vi "FetchIndividualElement.vi"() -> ()   [LabVIEW 2019]
uses:
  <vilib>/addons/database/Auxilliary.llb/DB Tools Cursor Type.ctl
  <vilib>/addons/database/Connection.llb/DB Tools Open Connec (String).vi
  <vilib>/addons/database/Connection.llb/Conn Execute.vi
  <vilib>/addons/database/Recordset.llb/Rec Fetch Integer Data (R).vi
  <vilib>/addons/database/Recordset.llb/Rec Fetch String Data (R).vi
  <vilib>/addons/database/Recordset.llb/Rec Destroy - Connection.vi
  <vilib>/addons/database/NI_Database_API.lvlib
panel:
  out "data 2":string
  out "?":i32
  in  "Tell Your ODBC server":string
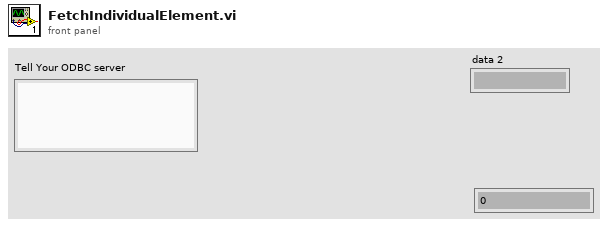
[diagram p1: front panel]
types:
  T1 = typedef "NI_Database_API.lvlib/DB Tools Cursor Type.ctl" = enum16{"forward-only", "keyset", "dynamic", "static"}
  T2 = typedef "NI_Database_API.lvlib/Conn ObjectReference.ctl" = refnum<k1>
  T3 = typedef "NI_Database_API.lvlib/Rec ObjectReference.ctl" = refnum<k1>
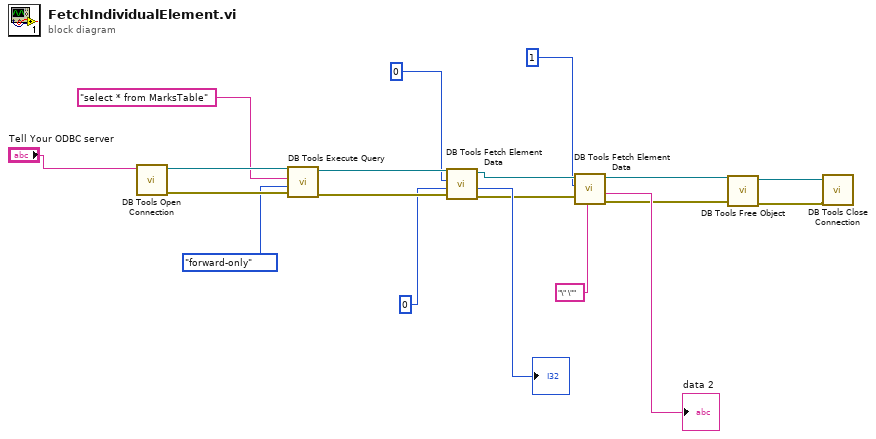
[diagram p0: block diagram]
diagram:
  n1 = call-poly <vilib>:"DB Tools Open Connection.vi"("connection information"="Tell Your ODBC server") -> ("error out"=w17:errorcluster, "connection reference"=w18:T2)  [unwired: 7 in]
  n2 = call-poly <vilib>:"DB Tools Execute Query.vi"("error in (no error)"=w17, "cursor type"=DB_Tools_Cursor_Type."forward-only", "SQL query"="select * from MarksTable", "connection reference"=w18) -> ("error out"=w14:errorcluster, "recordset reference"=w15:T3)  [unwired: 4 in]
  n3 = call-poly <vilib>:"DB Tools Fetch Element Data.vi"("error in (no error)"=w14, "type"=0, "column index"=0, "recordset reference"=w15) -> ("error out"=w9:errorcluster, "data"=→"?":i32, "recordset reference out"=w10:T3)  [unwired: 3 in]
  n4 = call-poly <vilib>:"DB Tools Fetch Element Data.vi"("error in (no error)"=w9, "type"="\" \"", "column index"=1, "recordset reference"=w10) -> ("error out"=w4:errorcluster, "data"=→"data 2":string, "recordset reference out"=w5:T3)  [unwired: 3 in]
  n5 = call-poly <vilib>:"DB Tools Free Object.vi"("error in (no error)"=w4, "recordset reference"=w5) -> ("error out"=w2:errorcluster, "connection reference"=w3:T2)  [unwired: 8 in]
  n6 = call <vilib>:"DB Tools Close Connection.vi"("error in (no error)"=w2, "connection reference"=w3) -> ()  [unwired: 5 in, 1 out]
